vi "Configure High Speed.vi"(0 "VISA resource name":refnum<visa-resource-name>, 1 "Enable High Speed Descrambling (F Disable)":bool, 2 "High Speed Serial Source (1: High Speed Source 1)":i32(ring)=1 items=["High Speed Source 1"=1, "High Speed Source 2"=2, "High Speed Source 3"=3, "High Speed Source 4"=4], 5 "Bus Channel (1: Serial Bus 1)":i32(ring)=1 items=["Serial Bus 1"=1, "Serial Bus 2"=2, "Serial Bus 3"=3, "Serial Bus 4"=4], 7 "Enable Idle (F: Disable)":bool, 9 "Display Format (1: Label)":i32(ring)=1 items=["K/D Code", "Label", "F8 Bit", "F10 Bit"], 11 "error in (no error)":errorcluster, 12 "High Speed Data Source (24: None)":i32(ring)=24 items=["Channel 1", "Channel 2", "Channel 3", "Channel 4", "Function 1", "Function 2", "Function 3", "Function 4", "Function 5", "Function 6", "Function 7", "Function 8", "Function 9", "Function 10", "Function 11", "Function 12", "Function 13", "Function 14", "Function 15", "Function 16", "Memory 1", "Memory 2", "Memory 3", "Memory 4", "None"]) -> (4 "VISA resource name out":refnum<visa-resource-name>, 15 "error out":errorcluster)   [LabVIEW 2020, in "Agilent 90000 Series.lvlib"]
doc: "Configures settings of high-speed serial bus.\n\n<b>Note:</b> \n1. This VI is new in firmware version 5.00.\n2. These commands are only valid when the high-speed (HS) serial decode type has been licensed and set with the :BUS:B<N>:TYPE command."
uses:
  Agilent 90000 Series.lvlib
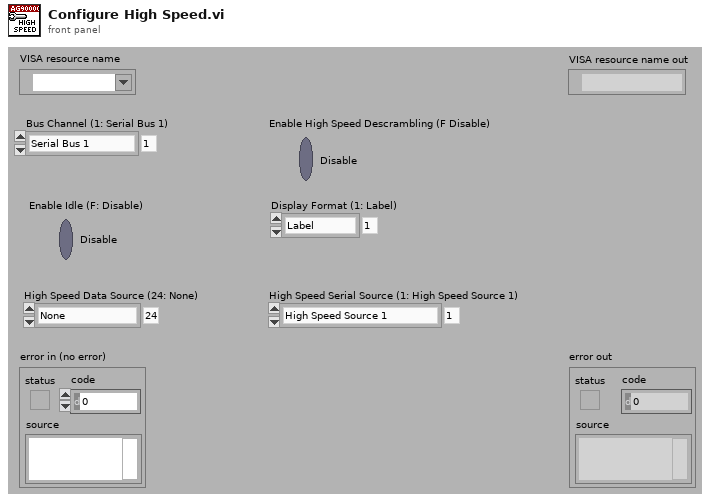
[diagram p1: front panel]
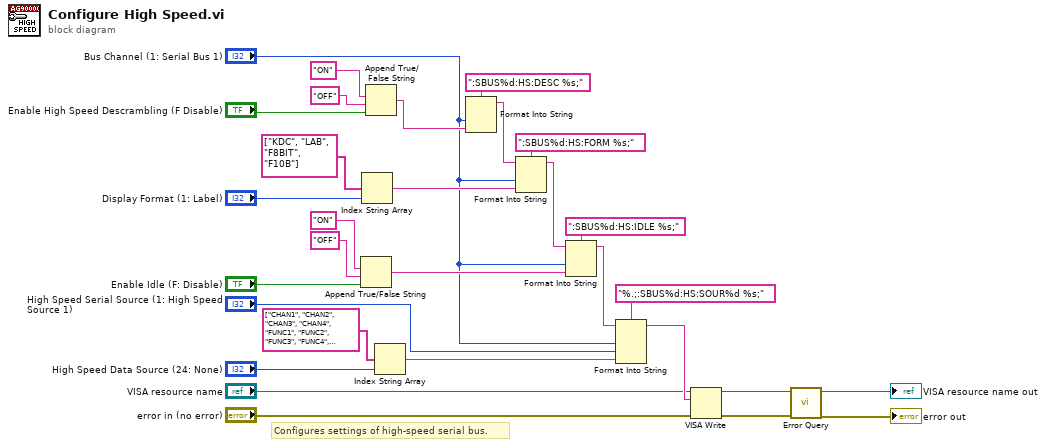
[diagram p0: block diagram]
diagram:
  # "Configures settings of high-speed serial bus."
  n1 = Append True/False String(1:"Enable Idle (F: Disable)", 2:"OFF", 3:"ON") -> (0:w20:string)  [unwired: 1 in]
  n2 = Index String Array(1:"Display Format (1: Label)", 2:string[] ["KDC", "LAB", "F8BIT", "F10B"] ("string array")) -> (0:w9:string)  [unwired: 1 in]
  n3 = Append True/False String(1:"Enable High Speed Descrambling (F Disable)", 2:"OFF", 3:"ON") -> (0:w26:string)  [unwired: 1 in]
  n4 = Index String Array(1:"High Speed Data Source (24: None)", 2:string[] ["CHAN1", "CHAN2", "CHAN3", "CHAN4", "FUNC1", "FUNC2", "FUNC3", "FUNC4", "FUNC5", "FUNC6", "FUNC7", "FUNC8", "FUNC9", "FUNC10", "FUNC11", "FUNC12", "FUNC13", "FUNC14", "FUNC15", "FUNC16", "WMEM1", "WMEM2", "WMEM3", "WMEM4", "NONE"] ("string array")) -> (0:w4:string)  [unwired: 1 in]
  n5 = Format Into String(format string=":SBUS%d:HS:DESC %s;", "Bus Channel (1: Serial Bus 1)", w26) -> (resulting string=w25:string)  [unwired: 2 in, 1 out]
  n6 = Format Into String(format string=":SBUS%d:HS:FORM %s;", initial string=w25, "Bus Channel (1: Serial Bus 1)", w9) -> (resulting string=w22:string)  [unwired: 1 in, 1 out]
  n7 = Format Into String(format string=":SBUS%d:HS:IDLE %s;", initial string=w22, "Bus Channel (1: Serial Bus 1)", w20) -> (resulting string=w19:string)  [unwired: 1 in, 1 out]
  n8 = Format Into String(format string="%.;:SBUS%d:HS:SOUR%d %s;", initial string=w19, "Bus Channel (1: Serial Bus 1)", "High Speed Serial Source (1: High Speed Source 1)", w4) -> (resulting string=w17:string)  [unwired: 1 in, 1 out]
  n9 = VISA Write(VISA resource name="VISA resource name", write buffer=w17, error in (no error)="error in (no error)") -> (VISA resource name out=w14:refnum<visa-resource-name>, error out=w13:errorcluster)  [unwired: 1 out]
  n10 = call "Error Query.vi"("error in (no error)"=w13, "VISA resource name"=w14) -> ("error out"=→"error out":errorcluster, "VISA resource name out"=→"VISA resource name out":refnum<visa-resource-name>)  [unwired: 6 in, 2 out]
